vi "Set Variables.vi"(8 "error in (no error)":errorcluster, 10 "Variables":variant, 11 "String Operations in":refnum<class "String Functions.lvclass">) -> (0 "error out":errorcluster, 3 "String Operations out":refnum<class "String Functions.lvclass">)   [LabVIEW 2019, in "String Functions.lvclass"]
uses:
  String Functions.lvclass
  String Functions.lvclass/String Functions.ctl
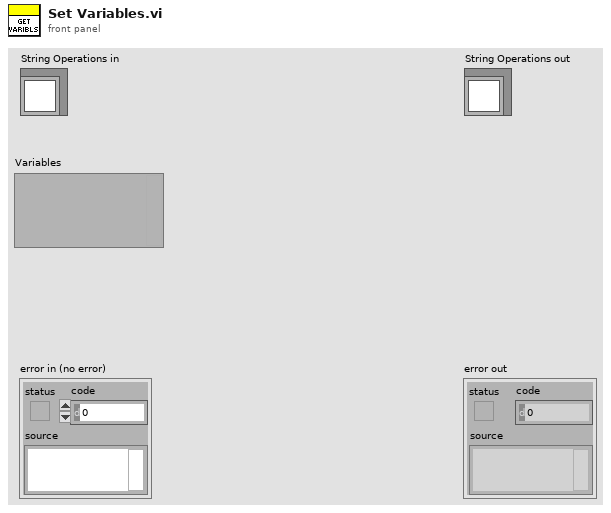
[diagram p1: front panel]
types:
  T1 = typedef "String Functions.lvclass/Variables.ctl" = cluster{"Str1":string, "Str2":string, "offset":i32, "length":i32, "num":dbl}
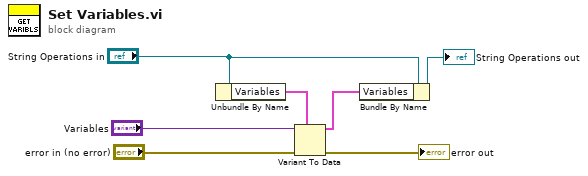
[diagram p0: block diagram]
diagram:
  n1 = Unbundle By Name("String Operations in") -> ("Variables"=w2:T1)
  n2 = Variant To Data(error in="error in (no error)", type=w2, Variant="Variables") -> (data=w1:T1, error out=→"error out":errorcluster)
  n3 = Bundle By Name(cluster="String Operations in", "Variables"=w1) -> (→"String Operations out":refnum<class "String Functions.lvclass">)
